vi "Fpga-OrderBook.vi"   [LabVIEW 2016]
uses:
  <vilib>/Platform/TimedLoop/XDataNode/timing_clust.ctl
  <vilib>/Platform/TimedLoop/XDataNode/nitl_modes.ctl
  <vilib>/Platform/TimedLoop/XDataNode/wakeup.ctl
  <vilib>/rvi/Emulation/niFpgaSctlEmulationGetInTimedLoop.vi
  <vilib>/rvi/Emulation/niFpgaEmulationReportErrorSimple.vi
  <vilib>/rvi/Emulation/niFpgaGetClockAttributes.vi
  <vilib>/rvi/Emulation/niFpgaCriticalErrorInLSC.vi
  <vilib>/rvi/DataTransferAndStorage/Container/Common/niFpgaContainerGetUniqueNameForEmu.vi
  <vilib>/rvi/DataTransferAndStorage/Container/Common/niFpgaContainerSetEmuInfo.vi
  <vilib>/rvi/eio/common/nirviEmuReportErrorAndStop.vi
  <vilib>/rvi/Emulation/niFpgaEmulationIsFPGAContextNoSignature.vi
  <vilib>/rvi/errors/niFpgaSetErrorForExecOnDevCompSimple.vi
  <vilib>/rvi/FIFO/Fifo_Resource/nirvififoEmulationSetSize.vi
  <vilib>/rvi/FIFO/Fifo_Resource/nirviFifoEmulationQueueMgr.vi
  <instcachedir>/0/nirviFifoEmulationQueueMgr_E5CAEC123FF24DC58D834DCA3CDAA9B5.lvgen/nirviFifoEmulationQueueMgr_E5CAEC123FF24DC58D834DCA3CDAA9B5_006.vi
  <vilib>/rvi/FIFO/Fifo_Resource/nirvififoEmulationDetermineInputValidOut.vi
  <vilib>/rvi/FIFO/Fifo_Resource/nirvififoEmulationCreateLock.vi
  <vilib>/rvi/Emulation/niFpgaProcessEmulError.vi
  <vilib>/rvi/FIFO/Fifo_Resource/nirvififoEmulationObtainLock.vi
  <vilib>/rvi/FIFO/Fifo_Resource/nirvififoEmulationReleaseLock.vi
  <vilib>/rvi/occurrence/nirviWaitOnOccurrenceBase.vi
  <vilib>/rvi/errors/nirviReportUnexpectedCaseInternalError.vi
  <vilib>/rvi/errors/nirviReportUnexpectedCaseInternalError (U32).vi
  <vilib>/rvi/DataTransferAndStorage/Container/Common/niFpgaContainerExecOnDevCompGetState.vi
  <vilib>/rvi/Memory/Memory_Emulation/niFpgaMemoryEmulationCacheClearOnFirstRun.vi
  <vilib>/rvi/Memory/Memory_Emulation/nirvimemoryEmulationManagerCache_MakeExclusive.vi
  <vilib>/rvi/Memory/Memory_Emulation/niFpgaMemoryEmulationValidateCache.vi
  <vilib>/rvi/Memory/Memory_Emulation/nirvimemoryEmulationManagerCache_InsertValue.vi
  <vilib>/Utility/error.llb/Clear Errors.vi
  <vilib>/rvi/Memory/Memory_Emulation/nirvimemoryEmulationManagerCache_ReleaseExclusive.vi
  <vilib>/rvi/Memory/Memory_Emulation/nirvimemoryEmulationManagerCache_GetValue.vi
  <vilib>/rvi/Memory/Memory_Emulation/nirvimemoryEmulationManagerCache_SetValue.vi
  <vilib>/rvi/Emulation/niFpgaSctlEmulationResourceMgr.vi
  <instcachedir>/0/nirviFifoEmulationQueueMgr_E5CAEC123FF24DC58D834DCA3CDAA9B5.lvgen/nirviFifoEmulationQueueMgr_E5CAEC123FF24DC58D834DCA3CDAA9B5_000.vi
  <vilib>/Platform/TimedLoop/XDataNode/XDataNode.xnode
  <vilib>/rvi/LocalResourceManager/LocalResourceManager.xnode
  <vilib>/rvi/DataTransferAndStorage/Container/XNode/niFpgaContainer.xnode
  <vilib>/rvi/FIFO/Fifo_Resource/nirvififoEmulationWrite.vi
  <vilib>/rvi/Memory/Memory_Emulation/niFpgaMemoryEmulationRefIn.vi
  <vilib>/rvi/FIFO/Fifo_Resource/nirvififoEmulationRead.vi
  <vilib>/Platform/TimedLoop/XDataNode/XDNodeRunTimeDep.lvlib
types:
  T1 = cluster{"Side":u16, "OrderRefNum":u64, "Price":u32, "Shares":u32}
  T2 = typedef "XDNodeRunTimeDep.lvlib/timing_clust.ctl" = cluster{"Expected End [f-1]":u64, "Actual End [f-1]":u64, "Finished Late? [f-1]":bool, "Expected End [i-1]":u64, "Actual End [i-1]":u64, "Finished Late? [i-1]":bool, "Expected Start [i]":u64, "Actual Start [i]":u64, "Expected Start [f]":u64, "Actual Start [f]":u64, "Source Name":string, "Structure Name":string, "Period":i64, "Deadline":i64, "Offset":i64, "Start":i64, "Priority":i32, "Timeout":i32, "Mode":T3, "Wakeup Reason":T4, "Error":errorcluster, "Source Type":string, "Secondary Source Type":string, "Global End Time":u64, "Global Start Time":u64, "Frame Duration":u64, "Iteration Duration":u64, "Assigned CPU":i32, "I/O Scan Engine Mode":u32}
  T3 = typedef "XDNodeRunTimeDep.lvlib/nitl_modes.ctl" = enum32{"No Change", "Process missed periods, maintain original phase", "Discard missed periods, maintain original phase", "Process missed periods, ignore original phase", "Discard missed periods, ignore original phase"}
  T4 = typedef "XDNodeRunTimeDep.lvlib/wakeup.ctl" = enum32{"Normal", "Aborted", "Asynchronous wakeup", "Timing source error", "Timed loop error", "Timeout"}
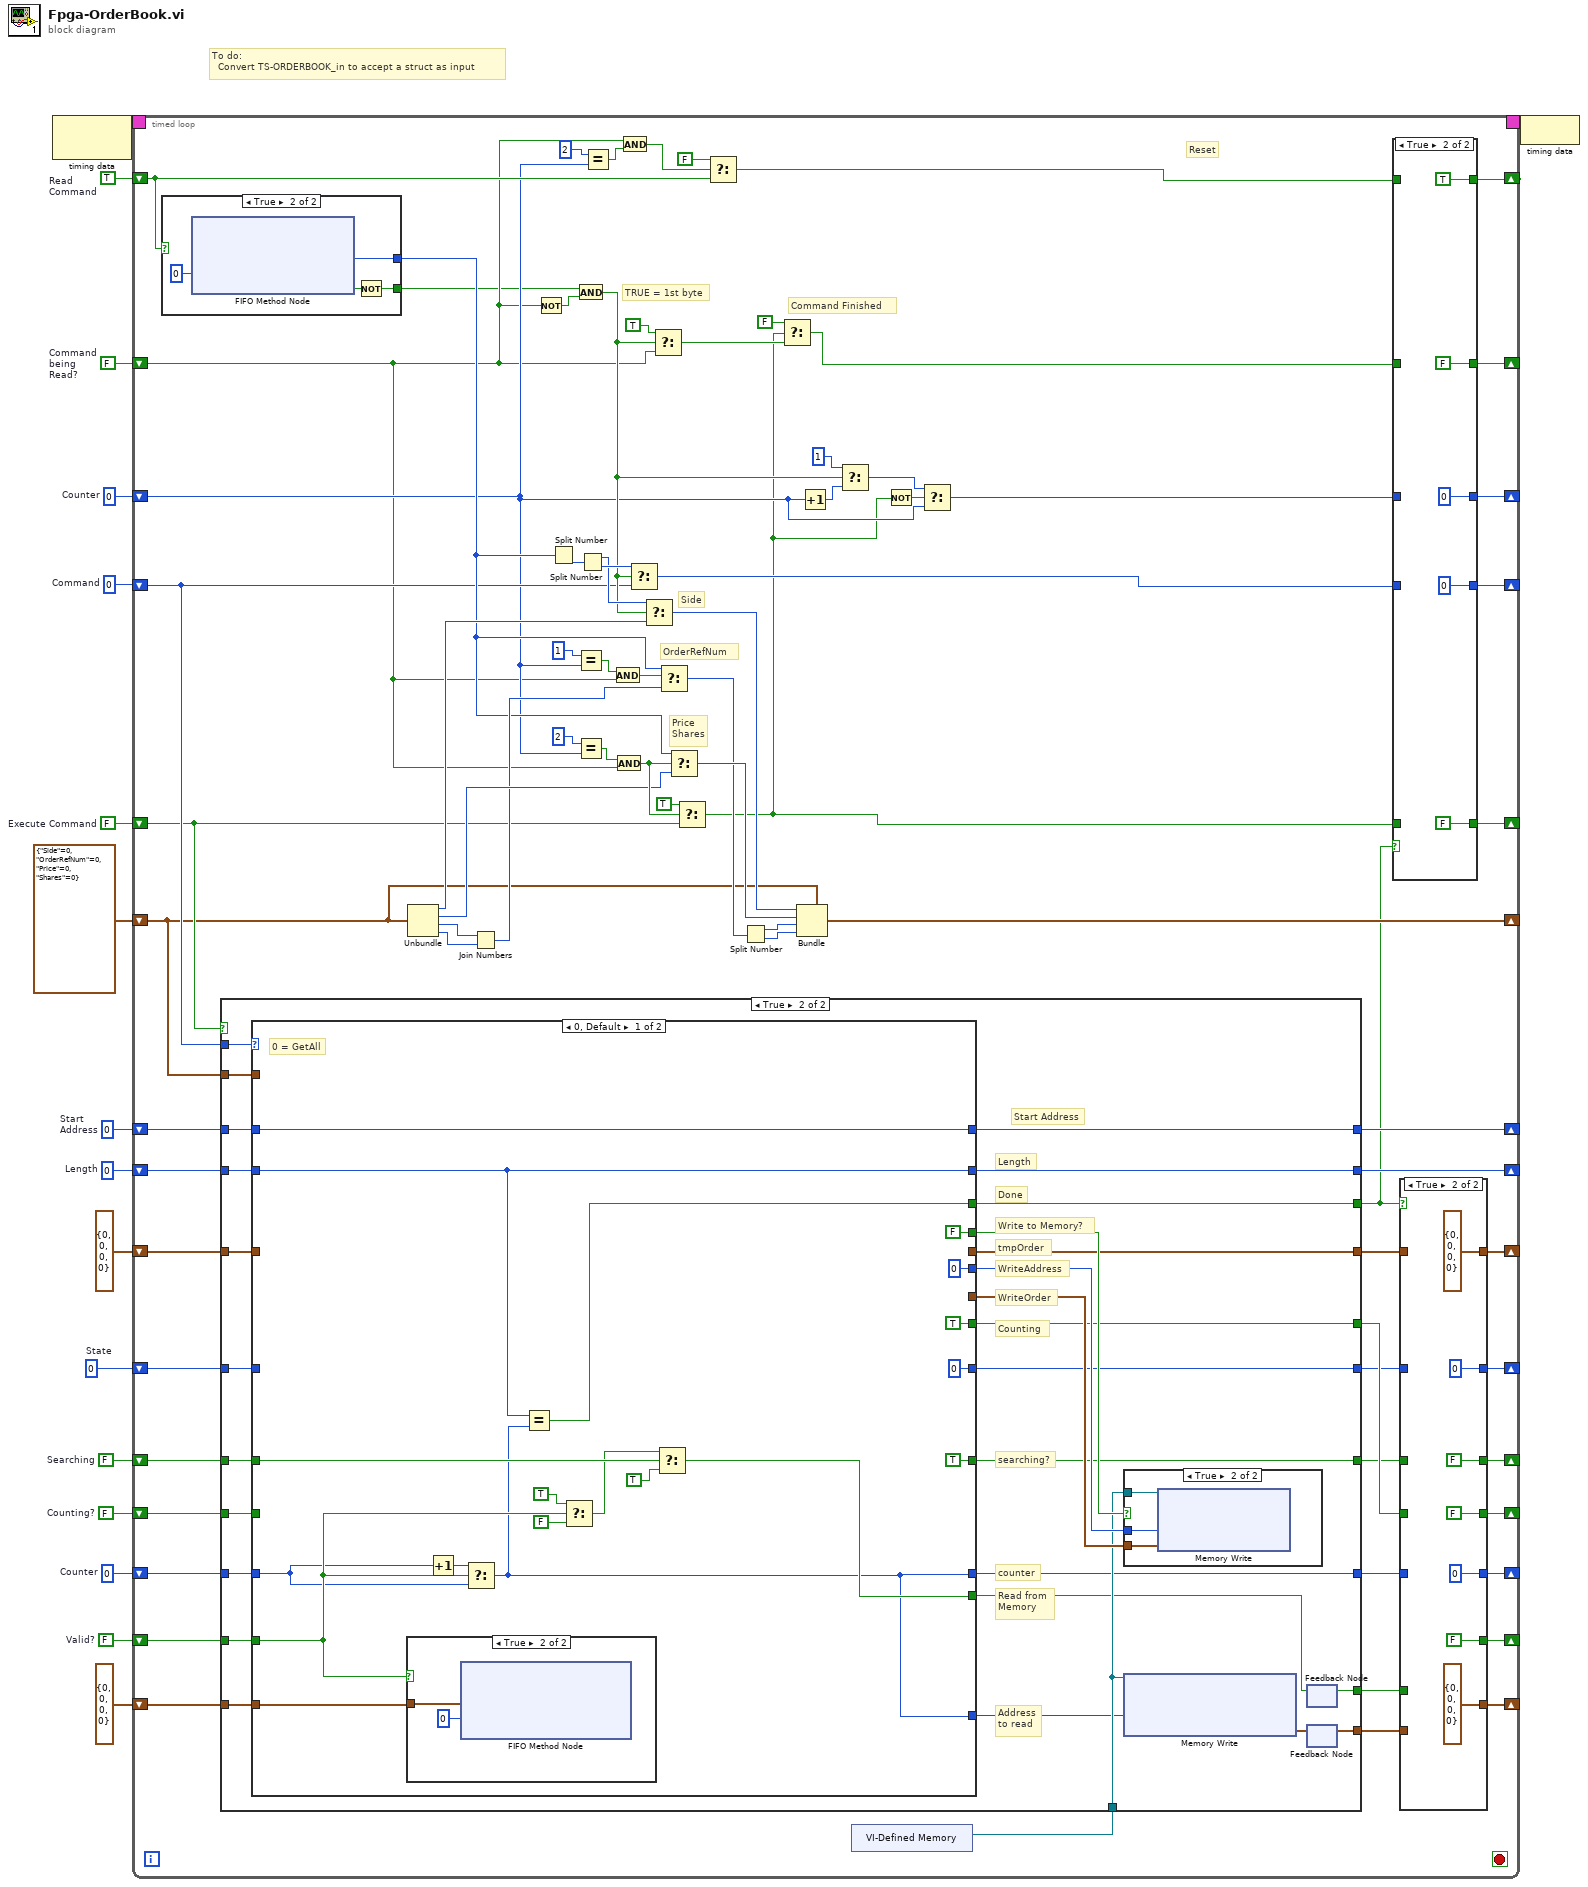
[diagram p0: block diagram]
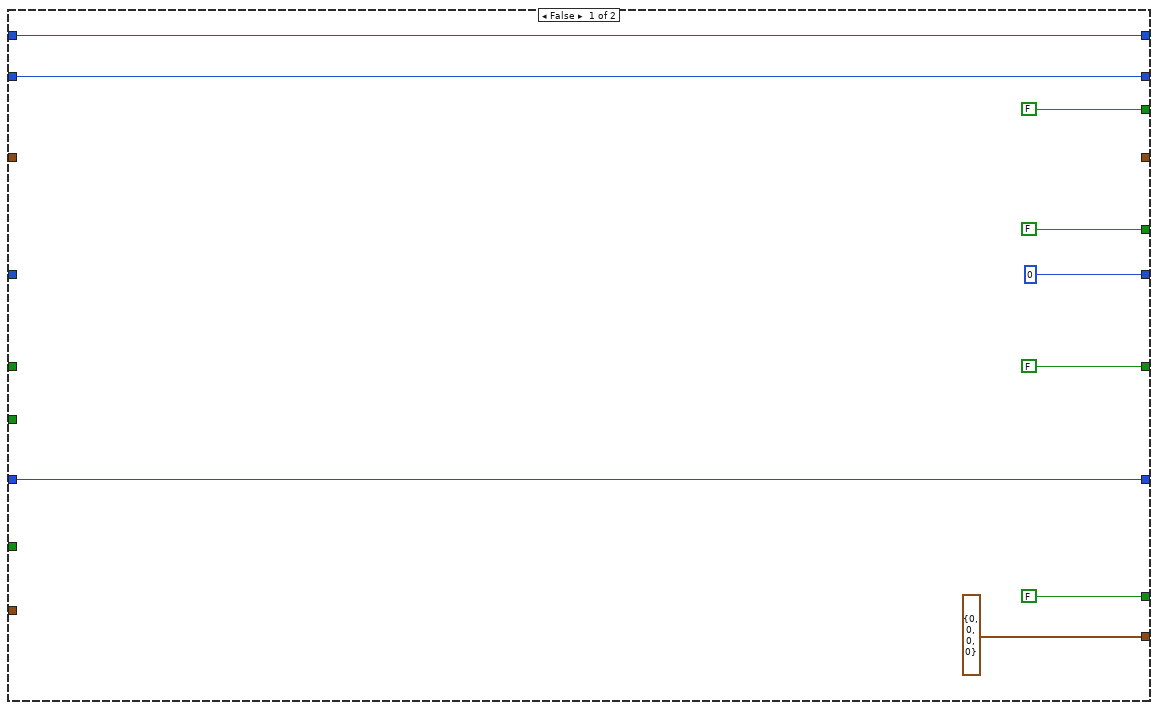
[diagram p4: hidden frame]
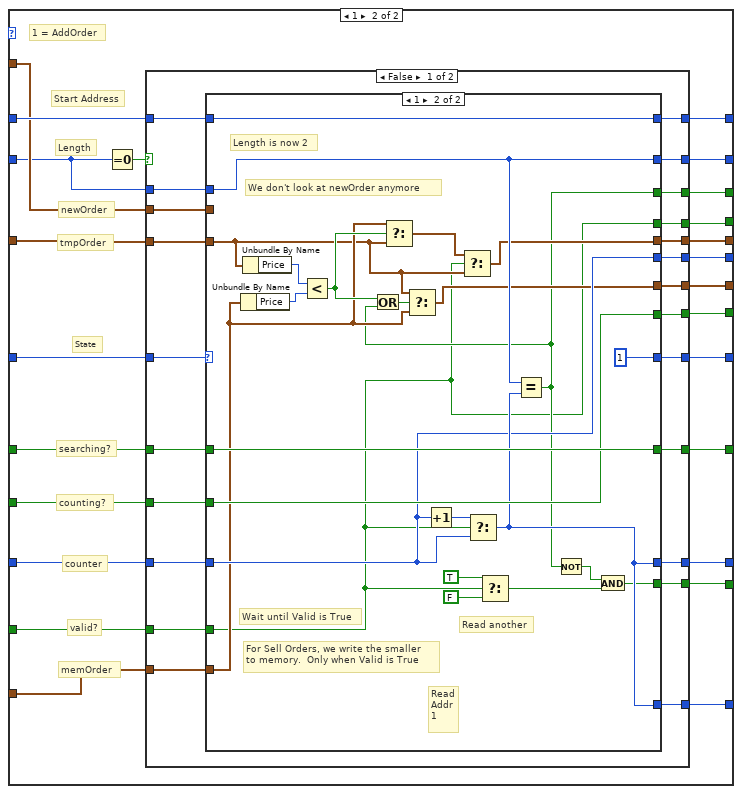
[diagram p7: hidden frame]
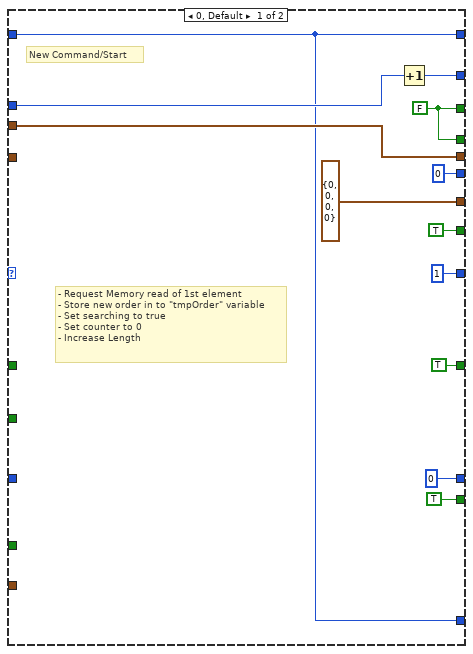
[diagram p8: hidden frame]
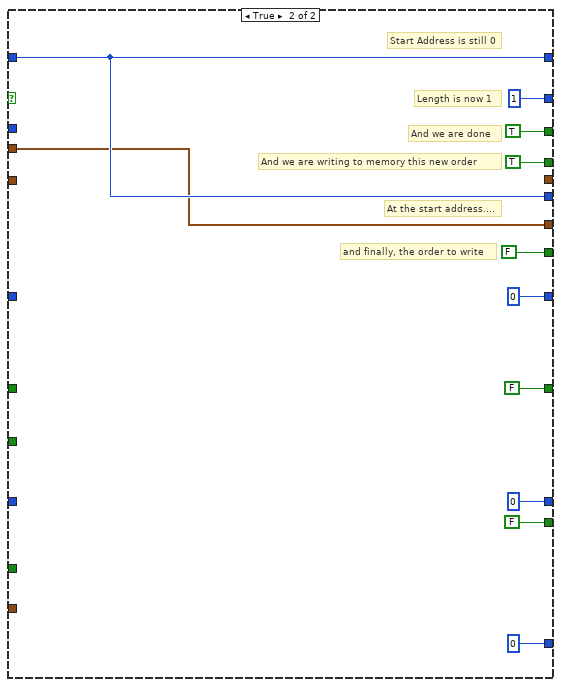
[diagram p9: hidden frame]
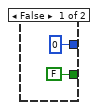
[diagram p10: hidden frame]
diagram:
  w1 = i16 0  # State
  w3 = FALSE  # Searching
  w5 = FALSE  # Valid?
  w6 = FALSE  # Counting?
  w8 = u64 0  # Counter
  w9 = FALSE  # Execute Command
  w11 = u64 0  # Length
  w10 = u64 0  # Start Address
  w12 = u64 0  # Counter
  w13 = u16 0  # Command
  w14 = FALSE  # Command being Read?
  w15 = TRUE  # Read Command
  # "To do:\n  Convert TS-ORDERBOOK_in to accept a struct as input"
  n1 = node-c288() -> (w17:T2)  [unwired: 1 in]
  n2 = timed-loop {
    timing: w17 -> [_]
    timing-out: [_] -> w16
    shift-right: [w49] -> _
    shift-left: w15 -> [w94]
    shift-right: [w48] -> _
    shift-left: w14 -> [w52]
    shift-right: [w45] -> _
    shift-left: w13 -> [w59]
    shift-right: [w47] -> _
    shift-left: w12 -> [w56]
    shift-right: [w87] -> _
    shift-left: w10 -> [w88]
    shift-right: [w89] -> _
    shift-left: w11 -> [w90]
    shift-right: [w43] -> _
    shift-left: w9 -> [w51]
    shift-right: [w33] -> _
    shift-left: w8 -> [w80]
    shift-right: [w74] -> _
    shift-left: T1 {"Side"=0, "OrderRefNum"=0, "Price"=0, "Shares"=0} ("Cluster") -> [w21]
    shift-right: [w36] -> _
    shift-left: w6 -> [w42]
    shift-right: [w27] -> _
    shift-left: T1 {"Side"=0, "OrderRefNum"=0, "Price"=0, "Shares"=0} ("Data") -> [w40]
    shift-right: [w28] -> _
    shift-left: w5 -> [w41]
    shift-right: [w35] -> _
    shift-left: w3 -> [w39]
    shift-right: [w31] -> _
    shift-left: T1 {"Side"=0, "OrderRefNum"=0, "Price"=0, "Shares"=0} ("Data") -> [w38]
    shift-right: [w24] -> _
    shift-left: w1 -> [w25]
    stop <- _ stop-if-true
    # "Command Finished"
    # "Reset"
    # "Price\nShares"
    # "OrderRefNum"
    # "Side"
    # "TRUE = 1st byte"
    n3 = case shown="True" w94 {
      tunnel: [FALSE ("Timed Out?") w278] -> w19
      tunnel: [u64 0 ("Element") w279] -> w61
      frame False {
      }
      frame True {
        n4 = xnode ("FIFO Method Node")("Timeout"=0) -> ("Element"=w279:u64, "Timed Out?"=w280:bool)  [unwired: 1 in, 1 out]
        n5 = Not(x=w280) -> (.not. x?=w278:bool)
      }
    }
    n6 = Unbundle(w21) -> ("Side"=w64:u16, "OrderRefNum"=w71:u64, "Price"=w67:u32, "Shares"=w66:u32)
    n7 = Join Numbers(hi=w67, lo=w66) -> ((hi.lo)=w62:u64)
    n8 = Not(x=w52) -> (.not. x?=w96:bool)
    n9 = Split Number(x=w61) -> (lo(x)=w73:u32)  [unwired: 1 out]
    n10 = And(x=w19, y=w96) -> (x .and. y?=w60:bool)
    n11 = Equal?(x=u64 1, y=w56) -> (x = y?=w53:bool)
    n12 = Equal?(x=u64 2, y=w56) -> (x = y?=w78:bool)
    n13 = Split Number(x=w73) -> (hi(x)=w63:u16, lo(x)=w65:u16)
    n14 = Equal?(x=u64 2, y=w56) -> (x = y?=w83:bool)
    n15 = And(x=w53, y=w52) -> (x .and. y?=w54:bool)
    n16 = And(x=w78, y=w52) -> (x .and. y?=w79:bool)
    n17 = And(x=w52, y=w83) -> (x .and. y?=w85:bool)
    n18 = Select(t=w65, s=w60, f=w59) -> (s? t:f=w44:u16)
    n19 = Select(t=w63, s=w60, f=w64) -> (s? t:f=w58:u16)
    n20 = Select(t=TRUE, s=w60, f=w52) -> (s? t:f=w76:bool)
    n21 = Select(t=w61, s=w54, f=w62) -> (s? t:f=w70:u64)
    n22 = Select(t=w61, s=w79, f=w71) -> (s? t:f=w72:u64)
    n23 = Select(t=TRUE, s=w79, f=w51) -> (s? t:f=w18:bool)
    n24 = Select(t=FALSE, s=w85, f=w94) -> (s? t:f=w50:bool)
    n25 = Split Number(x=w70) -> (hi(x)=w69:u32, lo(x)=w68:u32)
    n26 = Select(t=FALSE, s=w18, f=w76) -> (s? t:f=w20:bool)
    n27 = Bundle(cluster=w21, "Side"=w58, "OrderRefNum"=w72, "Price"=w69, "Shares"=w68) -> (w74:T1)
    n28 = Increment(x=w56) -> (x+1=w92:u64)
    n29 = Select(t=u64 1, s=w60, f=w92) -> (s? t:f=w55:u64)
    n30 = xnode "VI-Defined Memory"() -> ("Memory Out"=w75:refnum<k21>)
    n31 = case shown="True" w51 {
      tunnel: w59 -> [_ w157]
      tunnel: w90 -> [w129 w156]
      tunnel: [w129 w155] -> w89
      tunnel: w88 -> [w128 w153]
      tunnel: [w128 w154] -> w87
      tunnel: w80 -> [w126 w152]
      tunnel: [w126 w144] -> w32
      tunnel: [FALSE w151] -> w29
      tunnel: w75 -> [_ w145]
      tunnel: w21 -> [_ w140]
      tunnel: w42 -> [_ w147]
      tunnel: [FALSE w146] -> w37
      tunnel: [T1 {"Side"=0, "OrderRefNum"=0, "Price"=0, "Shares"=0} ("Data") w131] -> w26
      tunnel: [FALSE w132] -> w22
      tunnel: w41 -> [_ w142]
      tunnel: w40 -> [_ w141]
      tunnel: w39 -> [_ w139]
      tunnel: [FALSE w138] -> w34
      tunnel: w38 -> [_ w136]
      tunnel: [_ w135] -> w30
      tunnel: w25 -> [_ w134]
      tunnel: [i16 0 ("State") w133] -> w23
      frame False {
      }
      frame True {
        # "tmpOrder"
        # "searching?"
        # "counter"
        # "Read from\nMemory"
        # "Address\nto read"
        # "Counting"
        # "WriteOrder"
        # "WriteAddress"
        # "Write to Memory?"
        # "Length"
        # "Start Address"
        # "Done"
        n32 = case shown="0, Default" w157 {
          tunnel: w156 -> [w165 w183]
          tunnel: [w165 w205] -> w155
          tunnel: [w179 w203] -> w154
          tunnel: w153 -> [w179 w202]
          tunnel: w152 -> [w163 w194]
          tunnel: [w162 w193] -> w144
          tunnel: [w164 w201] -> w151
          tunnel: [FALSE w200] -> w150
          tunnel: w140 -> [_ w198]
          tunnel: [_ w197] -> w149
          tunnel: [u64 0 ("Start\nAddress") w199] -> w148
          tunnel: w147 -> [_ w196]
          tunnel: [TRUE ("Counting?") w195] -> w146
          tunnel: [w166 w189] -> w130
          tunnel: w142 -> [w172 w188]
          tunnel: w141 -> [w161 w187]
          tunnel: w139 -> [w169 w192]
          tunnel: [TRUE w191] -> w138
          tunnel: [w162 w190] -> w137
          tunnel: w136 -> [_ w186]
          tunnel: [_ w185] -> w135
          tunnel: w134 -> [_ w184]
          tunnel: [i16 0 ("State") w182] -> w133
          frame 0, Default {
            # "0 = GetAll"
            n33 = case shown="True" w172 {
              tunnel: w161 -> [_ w180]
              frame False {
              }
              frame True {
                n34 = xnode ("FIFO Method Node")("Element"=w180, "Timeout"=0) -> ()  [unwired: 1 in, 2 out]
              }
            }
            n35 = Increment(x=w163) -> (x+1=w173:u64)
            n36 = Select(t=w173, s=w172, f=w163) -> (s? t:f=w162:u64)
            n37 = Equal?(x=w165, y=w162) -> (x = y?=w164:bool)
            n38 = Select(t=TRUE, s=w172, f=FALSE) -> (s? t:f=w168:bool)
            n39 = Select(t=w168, s=w169, f=TRUE) -> (s? t:f=w166:bool)
          }
          frame 1 {
            # "State"
            # "Length"
            # "Start Address"
            # "memOrder"
            # "valid?"
            # "counter"
            # "counting?"
            # "searching?"
            # "tmpOrder"
            # "newOrder"
            # "1 = AddOrder"
            n40 = Equal To 0?(x=w183) -> (x = 0?=w204:bool)
            n41 = case shown="False" w204 {
              tunnel: [w227 u64 1 ("t")] -> w205
              tunnel: [w216 w272] -> w203
              tunnel: w202 -> [w215 w272]
              tunnel: [w223 TRUE] -> w201
              tunnel: [w222 TRUE] -> w200
              tunnel: [w221 w272] -> w199
              tunnel: w198 -> [w224 w271]
              tunnel: [w225 w271] -> w197
              tunnel: w196 -> [w206 _]
              tunnel: [w219 FALSE] -> w195
              tunnel: w194 -> [w208 _]
              tunnel: [w213 u64 0] -> w193
              tunnel: w192 -> [w207 _]
              tunnel: [w218 FALSE] -> w191
              tunnel: [w214 u64 0] -> w190
              tunnel: [w217 FALSE] -> w189
              tunnel: w188 -> [w211 _]
              tunnel: w187 -> [w209 _]
              tunnel: w186 -> [w210 _]
              tunnel: [w220 _] -> w185
              tunnel: w184 -> [w228 _]
              tunnel: w183 -> [w226 _]
              tunnel: [w212 i16 0 ("State")] -> w182
              frame False {
                n42 = case shown="1" w228 {
                  tunnel: [w229 w255] -> w227
                  tunnel: w226 -> [w240 w255]
                  tunnel: [T1 {"Side"=0, "OrderRefNum"=0, "Price"=0, "Shares"=0} ("Cluster") w251] -> w225
                  tunnel: w224 -> [w237 _]
                  tunnel: [w239 w243] -> w223
                  tunnel: [w239 w241] -> w222
                  tunnel: [u64 0 ("Start\nAddress") w254] -> w221
                  tunnel: [w237 w250] -> w220
                  tunnel: [TRUE w262] -> w219
                  tunnel: [TRUE w263] -> w218
                  tunnel: [TRUE w244] -> w217
                  tunnel: [w232 w264] -> w216
                  tunnel: w215 -> [w232 w264]
                  tunnel: [w232 w256] -> w214
                  tunnel: [u64 0 w256] -> w213
                  tunnel: [i16 1 ("State") i16 1 ("State")] -> w212
                  tunnel: w211 -> [_ w241]
                  tunnel: w210 -> [_ w245]
                  tunnel: w209 -> [_ w246]
                  tunnel: w208 -> [_ w254]
                  tunnel: w207 -> [_ w263]
                  tunnel: w206 -> [_ w262]
                  frame 0, Default {
                    w239 = FALSE
                    # "- Request Memory read of 1st element\n- Store new order in to \"tmpOrder\" variable\n- Set searching to true\n- Set counter to 0\n- Increase Length"
                    # "New Command/Start"
                    n43 = Increment(x=w240) -> (x+1=w229:u64)
                  }
                  frame 1 {
                    # "Read\nAddr\n1"
                    # "Read another"
                    # "Wait until Valid is True"
                    # "For Sell Orders, we write the smaller\nto memory.  Only when Valid is True"
                    # "We don't look at newOrder anymore"
                    # "Length is now 2"
                    n44 = Unbundle By Name(w246) -> ("Price"=w252:u32)
                    n45 = Unbundle By Name(w245) -> ("Price"=w253:u32)
                    n46 = Less?(x=w253, y=w252) -> (x < y?=w248:bool)
                    n47 = Select(t=w246, s=w248, f=w245) -> (s? t:f=w249:T1)
                    n48 = Increment(x=w254) -> (x+1=w258:u64)
                    n49 = Select(t=w249, s=w241, f=w245) -> (s? t:f=w250:T1)
                    n50 = Select(t=w258, s=w241, f=w254) -> (s? t:f=w256:u64)
                    n51 = Select(t=TRUE, s=w241, f=FALSE) -> (s? t:f=w261:bool)
                    n52 = Equal?(x=w255, y=w256) -> (x = y?=w243:bool)
                    n53 = Or(x=w248, y=w243) -> (x .or. y?=w247:bool)
                    n54 = Select(t=w245, s=w247, f=w246) -> (s? t:f=w251:T1)
                    n55 = Not(x=w243) -> (.not. x?=w242:bool)
                    n56 = And(x=w242, y=w261) -> (x .and. y?=w244:bool)
                  }
                }
              }
              frame True {
                # "and finally, the order to write"
                # "At the start address...."
                # "And we are writing to memory this new order"
                # "And we are done"
                # "Length is now 1"
                # "Start Address is still 0"
              }
            }
          }
        }
        n57 = case shown="True" w150 {
          tunnel: w145 -> [_ w160]
          tunnel: w149 -> [_ w159]
          tunnel: w148 -> [_ w158]
          frame False {
          }
          frame True {
            n58 = xnode ("Memory Write")("Address"=w158, "Data"=w159, "Memory In"=w160) -> ()  [unwired: 1 out]
          }
        }
        n59 = xnode ("Memory Write")("Address"=w137, "Memory In"=w145) -> ("Data"=w143:T1)  [unwired: 1 out]
        n60 = feedback-in #1(w130) -> ()
        n61 = feedback #1() -> (w132:bool)  [unwired: 1 in]
        n62 = feedback-in #2(w143) -> ()
        n63 = feedback #2() -> (w131:T1)  [unwired: 1 in]
      }
    }
    n64 = Not(x=w18) -> (.not. x?=w57:bool)
    n65 = Select(t=w55, s=w57, f=w56) -> (s? t:f=w46:u64)
    n66 = case shown="True" w29 {
      tunnel: w50 -> [w115 _]
      tunnel: [w115 TRUE ("Read\nCommand")] -> w49
      tunnel: [w114 FALSE ("Command\nbeing\nRead?")] -> w48
      tunnel: w20 -> [w114 _]
      tunnel: [w113 u64 0 ("Counter")] -> w47
      tunnel: w46 -> [w113 _]
      tunnel: [w112 u16 0 ("Command")] -> w45
      tunnel: w44 -> [w112 _]
      tunnel: [w111 FALSE ("Execute Command")] -> w43
      tunnel: w18 -> [w111 _]
      frame False {
      }
      frame True {
      }
    }
    n67 = case shown="True" w29 {
      tunnel: w37 -> [w103 _]
      tunnel: [w103 FALSE ("Counting?")] -> w36
      tunnel: [w102 FALSE] -> w35
      tunnel: w34 -> [w102 _]
      tunnel: [w101 u64 0 ("Counter")] -> w33
      tunnel: w32 -> [w101 _]
      tunnel: [w100 T1 {"Side"=0, "OrderRefNum"=0, "Price"=0, "Shares"=0} ("Cluster")] -> w31
      tunnel: w30 -> [w100 _]
      tunnel: [w99 FALSE] -> w28
      tunnel: w22 -> [w99 _]
      tunnel: [w98 T1 {"Side"=0, "OrderRefNum"=0, "Price"=0, "Shares"=0} ("Data")] -> w27
      tunnel: w26 -> [w98 _]
      tunnel: [w97 i16 0 ("State")] -> w24
      tunnel: w23 -> [w97 _]
      frame False {
      }
      frame True {
      }
    }
  }
  n68 = node-c288(w16) -> ()
